vi "Recieve Response with Result.vi"(4 "Finished":bool=TRUE, 6 "Result":refnum<class "Mag Lab Result.lvclass">, 8 "error in (no error)":errorcluster, 9 "Requestor":string, 10 "Requestee":string, 11 "Meter Measurement in":refnum<class "Meter Measurement.lvclass">) -> (0 "error out":errorcluster, 3 "Meter Measurement out":refnum<class "Meter Measurement.lvclass">)   [LabVIEW 2015, in "Meter Measurement.lvclass"]
uses:
  Meter Measurement.lvclass
  Mag Lab Result/Mag Lab Result.lvclass
  Mag Lab Root/Mag Lab Root.lvclass/Mag Lab Root.ctl
  Meter Measurement.lvclass/Meter Measurement.ctl
  <vilib>/ActorFramework/Actor/Actor.lvclass/Actor.ctl
  Mag Lab Root Messages/Recieve Response with Result Msg/Recieve Response with Result Msg.lvclass/Recieve Response with Result Msg.ctl
  <vilib>/ActorFramework/Message Enqueuer/Message Enqueuer.lvclass/Message Enqueuer.ctl
  <vilib>/ActorFramework/Message Enqueuer/Enqueue.vi
  <vilib>/ActorFramework/Message Priority Queue/Priority Enqueue.vi
  Mag Lab Root Messages/Recieve Response with Result Msg/Recieve Response with Result Msg.lvclass
  Mag Lab Root/Mag Lab Root.lvclass
  <vilib>/ActorFramework/Actor/Actor.lvclass
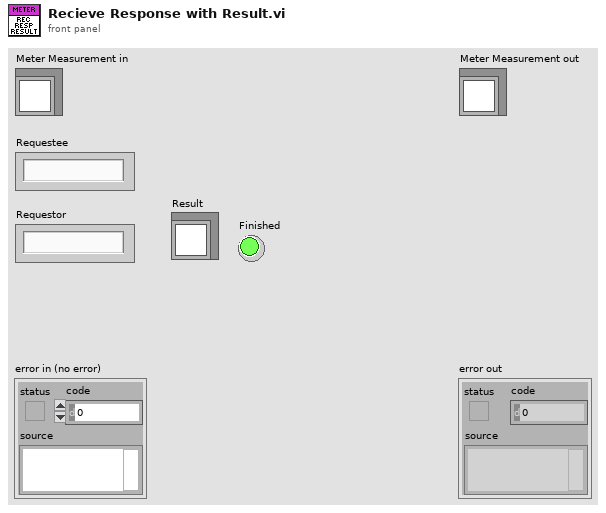
[diagram p1: front panel]
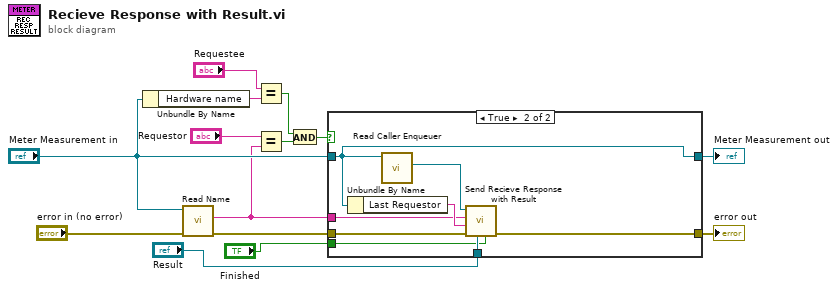
[diagram p0: block diagram]
diagram:
  n1 = Unbundle By Name("Meter Measurement in") -> ("Hardware name"=w13:string)
  n2 = call "Read Name.vi"("error in (no error)"="error in (no error)", "Mag Lab Root in"="Meter Measurement in") -> ("error out"=w8:errorcluster, "Name"=w4:string)  [unwired: 7 in, 1 out]
  n3 = Equal?(x="Requestee", y=w13) -> (x = y?=w12:bool)
  n4 = Equal?(x="Requestor", y=w4) -> (x = y?=w11:bool)
  n5 = And(x=w12, y=w11) -> (x .and. y?=w10:bool)
  n6 = case shown="True" w10 {
    tunnel: "Meter Measurement in" -> [w15 w19]
    tunnel: w4 -> [_ w21]
    tunnel: w8 -> [w16 w24]
    tunnel: [w16 w20] -> w6
    tunnel: [w15 w19] -> w5
    tunnel: "Result" -> [_ w18]
    tunnel: "Finished" -> [_ w17]
    frame False {
    }
    frame True {
      n7 = Unbundle By Name(w19) -> ("Last Requestor"=w22:string)
      n8 = call <vilib>:"Read Caller Enqueuer.vi"("Actor"=w19) -> ("Caller Enqueuer"=w23:refnum<class "Message Enqueuer.lvclass">)  [unwired: 10 in]
      n9 = call "Send Recieve Response with Result.vi"("Finished"=w17, "Result"=w18, "error in (no error)"=w24, "Requestor"=w22, "Requestee"=w21, "Message Enqueuer"=w23) -> ("error out"=w20:errorcluster)  [unwired: 4 in, 1 out]
    }
  }
  "error out" <- w6
  "Meter Measurement out" <- w5
